vi "Write Power DVR FIFO.vi"(6 "FIFO Timestamps":T1, 8 "error in (no error)":errorcluster, 9 "Timeout (ms)":i32=100, 10 "Data In":refnum<data-value>[](array[refnum]), 11 "CIFTag in":refnum<class "CIF_NIChn_Fifo_Power_DVR.lvclass">) -> (0 "error out":errorcluster, 1 "timed out?":bool, 2 "Data Out":refnum<data-value>[](array[refnum]), 3 "CIFTag out":refnum<class "CIF_NIChn_Fifo_Power_DVR.lvclass">)   [LabVIEW 2021, in "CIF_NIChn_Fifo_Power_DVR.lvclass"]
uses:
  CIF_NIChn_Fifo_Power_DVR.lvclass
  CIF_NIChn_Fifo_Power_DVR.lvclass/CIF_NIChn_Fifo_Power_DVR.ctl
  NIChn/CIF_NIChn.lvclass
  <vilib>/CIFChannels/CIFChannelCore.lvlib
  D:/dev/CIF-LVCore/src/Channels/CIF_NIChn/NIChn/CIF_NIChn.lvclass
  D:/dev/CIF-LVCore/src/Channels/CIFChannels/CIFChannels.lvclass
  D:/dev/CIF-LVCore/src/Channels/CIF_NIChn/FIFO_Power_DVR/CIF_NIChn_Fifo_Power_DVR.lvclass
  ChannelCommon/CIFFIFO/CIFfifo.lvclass
  ChannelCommon/typedef/TimeStamps.ctl
  ChannelCommon/ChannelCommon.lvlib
  ChannelCommon/typedef/Datatype Waveform.ctl
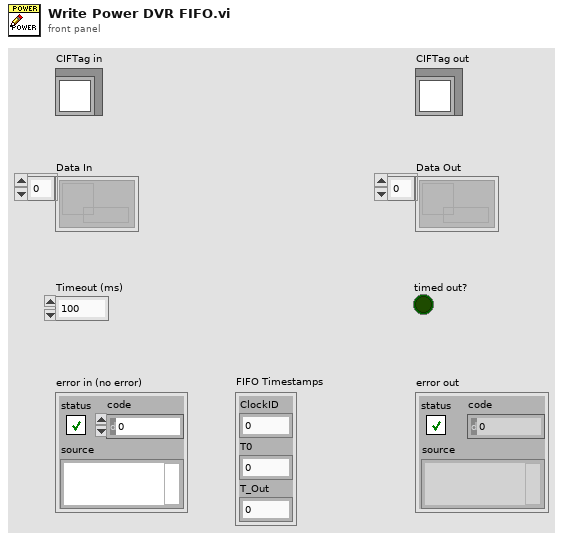
[diagram p1: front panel]
types:
  T1 = typedef "ChannelCommon.lvlib/TimeStamps.ctl" = cluster{"ClockID":u8, "T0":u64, "T_Out":u64}
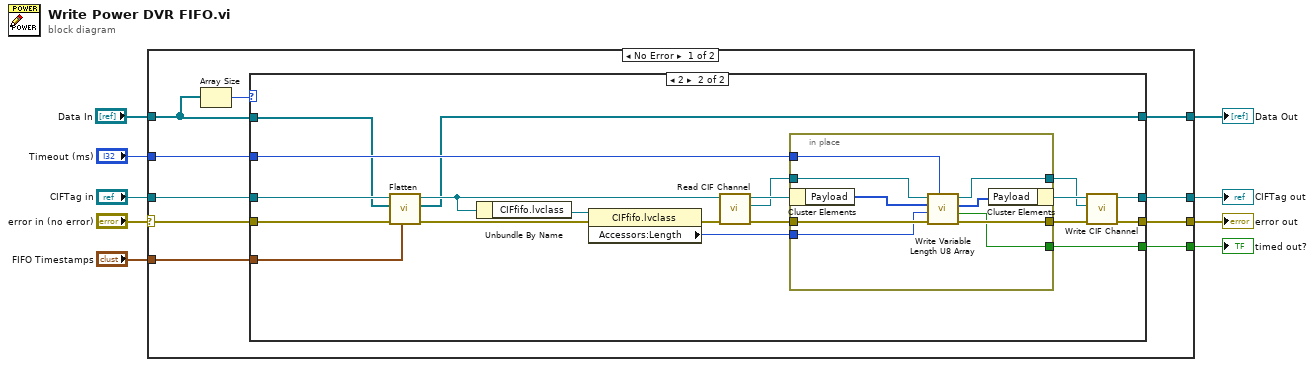
[diagram p0: block diagram]
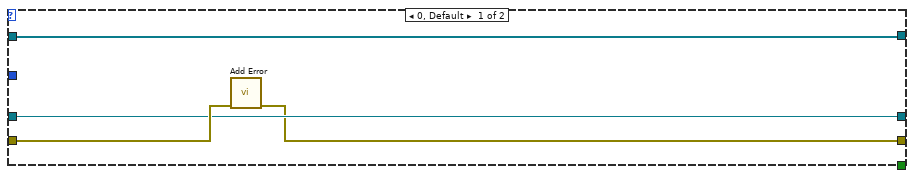
[diagram p2: hidden frame]
diagram:
  n1 = case shown="No Error" "error in (no error)" {
    selector: "error in (no error)" -> [w14 w55]
    tunnel: [w16 w55] -> w8
    tunnel: [w18 w54] -> w6
    tunnel: "CIFTag in" -> [w15 w54]
    tunnel: [w19 _] -> w5
    tunnel: "Timeout (ms)" -> [w17 _]
    tunnel: [w13 w53] -> w1
    tunnel: "Data In" -> [w12 w53]
    tunnel: "FIFO Timestamps" -> [w10 _]
    frame No Error {
      n2 = Array Size(array=w12) -> (size(s)=w11:i32)
      n3 = case shown="2" w11 {
        tunnel: [_ w43] -> w19
        tunnel: [w22 w39] -> w18
        tunnel: w17 -> [_ w35]
        tunnel: [w21 w34] -> w16
        tunnel: w15 -> [w22 w31]
        tunnel: w14 -> [w23 w28]
        tunnel: [w20 w26] -> w13
        tunnel: w12 -> [w20 w25]
        tunnel: w10 -> [_ w24]
        frame 0, Default {
          n4 = call "Add Error.vi"("error in (no error)"=w23) -> ("error out"=w21:errorcluster)  [unwired: 10 in]
        }
        frame 2 {
          n5 = call "Flatten.vi"("FIFO Timestamps"=w24, "error in (no error)"=w28, "Data In"=w25, "CIFTag in"=w31) -> ("error out"=w29:errorcluster, "Data Out"=w26:refnum<data-value>[], "CIFTag out"=w30:refnum<class "CIF_NIChn_Fifo_Power_DVR.lvclass">)  [unwired: 5 in]
          n6 = Unbundle By Name(w30) -> ("CIFfifo.lvclass"=w33:refnum<class "CIFfifo.lvclass">)
          n7 = property class="CIFfifo.lvclass"(reference=w33, error in=w29) -> (error out=w32:errorcluster, "Accessors:Length"=w27:u64)  [unwired: 1 out]
          n8 = call "Read CIF Channel.vi"("error in (no error)"=w32, "CIFTag in"=w30) -> ("error out"=w41:errorcluster, "CIF Channel"=w37:refnum<k21>, "CIFTag out"=w42:refnum<class "CIF_NIChn_Fifo_Power_DVR.lvclass">)  [unwired: 7 in]
          n9 = in-place {
            in-place-border: w41 -> [w52]
            in-place-border: [w51] -> w38
            in-place-border: [w50] -> w43
            in-place-border: w37 -> [w49]
            in-place-border: [w48] -> w36
            in-place-border: w35 -> [w47]
            in-place-border: w27 -> [w45]
            n10 = in-place-cluster #1(w42) -> ("Payload"=w46:u8[])
            n11 = call <vilib>:"Write Variable Length U8 Array.vi"("Timeout (ms)"=w47, "error in"=w52, "numElements"=w45, "U8 Array in"=w46, "CIF Channel in"=w49) -> ("error out"=w51:errorcluster, "Timed out?"=w50:bool, "U8 Array out"=w44:u8[], "CIF Channel out"=w48:refnum<k21>)  [unwired: 3 in]
            n12 = in-place-cluster #1("Payload"=w44) -> (w40:refnum<class "CIF_NIChn_Fifo_Power_DVR.lvclass">)
          }
          n13 = call "Write CIF Channel.vi"("error in (no error)"=w38, "CIF Channel"=w36, "CIFTag in"=w40) -> ("error out"=w34:errorcluster, "CIFTag out"=w39:refnum<class "CIF_NIChn_Fifo_Power_DVR.lvclass">)  [unwired: 7 in]
        }
      }
    }
    frame Error {
    }
  }
  "error out" <- w8
  "CIFTag out" <- w6
  "timed out?" <- w5
  "Data Out" <- w1
